vi "VerifyAcqIdle.vi"(8 "error in (no error)":errorcluster, 11 "S4GUI in":refnum<class "S4GUI.lvclass">) -> (0 "error out":errorcluster, 2 "idle":bool, 3 "S4GUI out":refnum<class "S4GUI.lvclass">)   [LabVIEW 2018, in "S4GUI.lvclass"]
uses:
  S4GUI.lvclass
  S4GUI.lvclass/S4GUI.ctl
  Acquisition/Acquisition.lvclass
  Channel/Channel.lvclass
  StateMachine/State Machine.lvclass
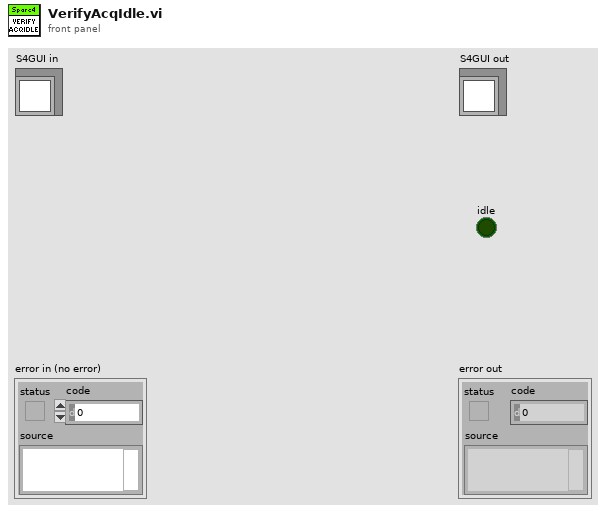
[diagram p1: front panel]
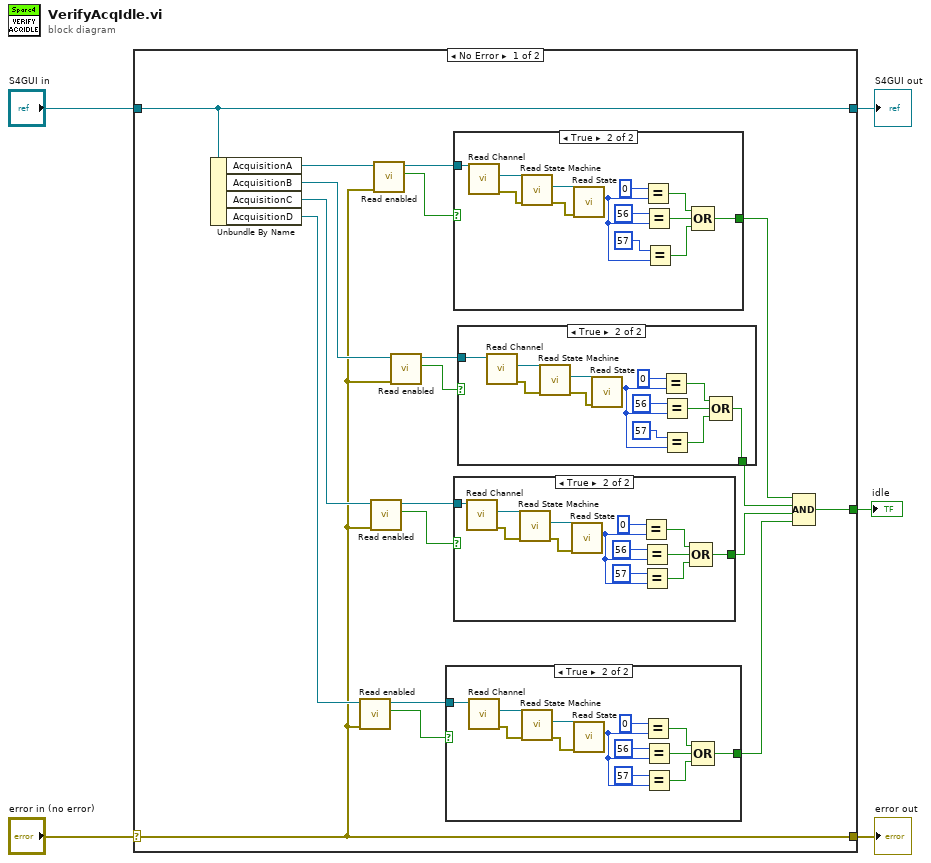
[diagram p0: block diagram]
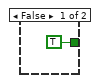
[diagram p2: hidden frame]
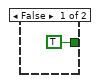
[diagram p3: hidden frame]
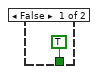
[diagram p4: hidden frame]
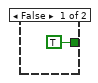
[diagram p5: hidden frame]
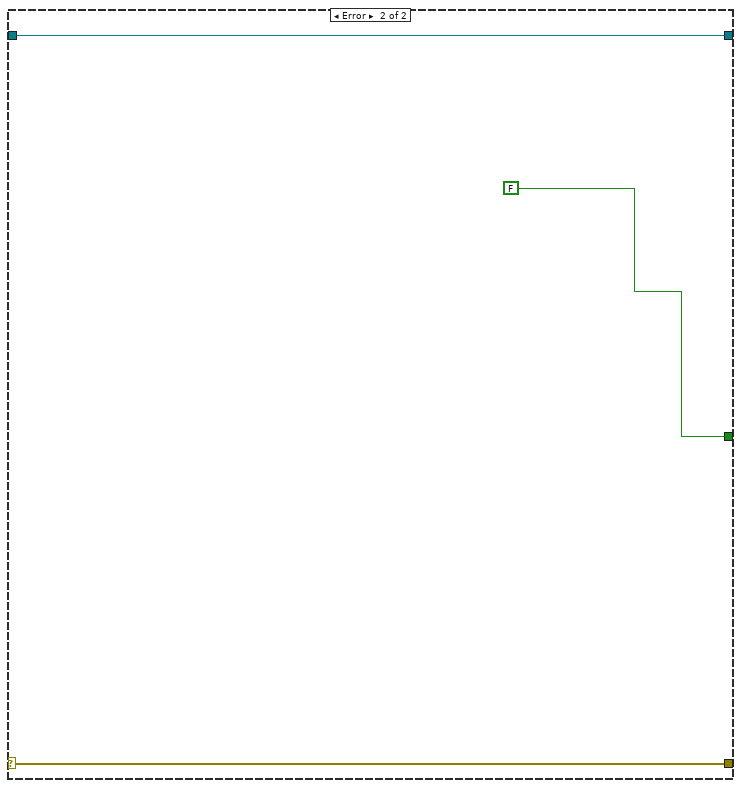
[diagram p6: hidden frame]
diagram:
  n1 = case shown="No Error" "error in (no error)" {
    selector: "error in (no error)" -> [w6 w83]
    tunnel: [w6 w83] -> w4
    tunnel: [w24 w82] -> w2
    tunnel: "S4GUI in" -> [w24 w82]
    tunnel: [w19 FALSE] -> w1
    frame No Error {
      n2 = Unbundle By Name(w24) -> ("AcquisitionA"=w18:refnum<class "Acquisition.lvclass">, "AcquisitionB"=w15:refnum<class "Acquisition.lvclass">, "AcquisitionC"=w12:refnum<class "Acquisition.lvclass">, "AcquisitionD"=w9:refnum<class "Acquisition.lvclass">)
      n3 = call-dynamic "Read enabled.vi"("error in (no error)"=w6, "Server in"=w9) -> ("enabled"=w7:bool, "Server out"=w8:refnum<class "Acquisition.lvclass">)  [unwired: 7 in, 1 out]
      n4 = call-dynamic "Read enabled.vi"("error in (no error)"=w6, "Server in"=w12) -> ("enabled"=w10:bool, "Server out"=w11:refnum<class "Acquisition.lvclass">)  [unwired: 7 in, 1 out]
      n5 = call-dynamic "Read enabled.vi"("error in (no error)"=w6, "Server in"=w18) -> ("enabled"=w16:bool, "Server out"=w17:refnum<class "Acquisition.lvclass">)  [unwired: 7 in, 1 out]
      n6 = call-dynamic "Read enabled.vi"("error in (no error)"=w6, "Server in"=w15) -> ("enabled"=w13:bool, "Server out"=w14:refnum<class "Acquisition.lvclass">)  [unwired: 7 in, 1 out]
      n7 = case shown="True" w7 {
        tunnel: w8 -> [_ w29]
        tunnel: [TRUE w28] -> w20
        frame False {
        }
        frame True {
          n8 = call-dynamic "Read Channel.vi"("Acquisition in"=w29) -> ("error out"=w27:errorcluster, "Channel.lvclass"=w34:refnum<class "Channel.lvclass">)  [unwired: 8 in, 1 out]
          n9 = call-dynamic "Read State Machine.vi"("error in (no error)"=w27, "Device in"=w34) -> ("error out"=w26:errorcluster, "State Machine.lvclass"=w33:refnum<class "State Machine.lvclass">)  [unwired: 7 in, 1 out]
          n10 = call-dynamic "Read State.vi"("error in (no error)"=w26, "State Machine in"=w33) -> ("State"=w32:i32)  [unwired: 7 in, 2 out]
          n11 = Equal?(x=0, y=w32) -> (x = y?=w37:bool)
          n12 = Equal?(x=56, y=w32) -> (x = y?=w36:bool)
          n13 = Equal?(x=57, y=w32) -> (x = y?=w35:bool)
          n14 = Compound Arithmetic op=OR(w37, w36, w35) -> (w28:bool)
        }
      }
      n15 = case shown="True" w16 {
        tunnel: [TRUE w76] -> w23
        tunnel: w17 -> [_ w75]
        frame False {
        }
        frame True {
          n16 = call-dynamic "Read Channel.vi"("Acquisition in"=w75) -> ("error out"=w69:errorcluster, "Channel.lvclass"=w74:refnum<class "Channel.lvclass">)  [unwired: 8 in, 1 out]
          n17 = call-dynamic "Read State Machine.vi"("error in (no error)"=w69, "Device in"=w74) -> ("error out"=w68:errorcluster, "State Machine.lvclass"=w73:refnum<class "State Machine.lvclass">)  [unwired: 7 in, 1 out]
          n18 = call-dynamic "Read State.vi"("error in (no error)"=w68, "State Machine in"=w73) -> ("State"=w72:i32)  [unwired: 7 in, 2 out]
          n19 = Equal?(x=0, y=w72) -> (x = y?=w79:bool)
          n20 = Equal?(x=56, y=w72) -> (x = y?=w78:bool)
          n21 = Equal?(x=57, y=w72) -> (x = y?=w77:bool)
          n22 = Compound Arithmetic op=OR(w79, w78, w77) -> (w76:bool)
        }
      }
      n23 = case shown="True" w10 {
        tunnel: w11 -> [_ w43]
        tunnel: [TRUE w42] -> w21
        frame False {
        }
        frame True {
          n24 = call-dynamic "Read Channel.vi"("Acquisition in"=w43) -> ("error out"=w41:errorcluster, "Channel.lvclass"=w48:refnum<class "Channel.lvclass">)  [unwired: 8 in, 1 out]
          n25 = call-dynamic "Read State Machine.vi"("error in (no error)"=w41, "Device in"=w48) -> ("error out"=w40:errorcluster, "State Machine.lvclass"=w47:refnum<class "State Machine.lvclass">)  [unwired: 7 in, 1 out]
          n26 = call-dynamic "Read State.vi"("error in (no error)"=w40, "State Machine in"=w47) -> ("State"=w46:i32)  [unwired: 7 in, 2 out]
          n27 = Equal?(x=0, y=w46) -> (x = y?=w51:bool)
          n28 = Equal?(x=56, y=w46) -> (x = y?=w50:bool)
          n29 = Equal?(x=57, y=w46) -> (x = y?=w49:bool)
          n30 = Compound Arithmetic op=OR(w51, w50, w49) -> (w42:bool)
        }
      }
      n31 = case shown="True" w13 {
        tunnel: w14 -> [_ w57]
        tunnel: [TRUE w56] -> w22
        frame False {
        }
        frame True {
          n32 = call-dynamic "Read Channel.vi"("Acquisition in"=w57) -> ("error out"=w55:errorcluster, "Channel.lvclass"=w62:refnum<class "Channel.lvclass">)  [unwired: 8 in, 1 out]
          n33 = call-dynamic "Read State Machine.vi"("error in (no error)"=w55, "Device in"=w62) -> ("error out"=w54:errorcluster, "State Machine.lvclass"=w61:refnum<class "State Machine.lvclass">)  [unwired: 7 in, 1 out]
          n34 = call-dynamic "Read State.vi"("error in (no error)"=w54, "State Machine in"=w61) -> ("State"=w60:i32)  [unwired: 7 in, 2 out]
          n35 = Equal?(x=0, y=w60) -> (x = y?=w65:bool)
          n36 = Equal?(x=56, y=w60) -> (x = y?=w64:bool)
          n37 = Equal?(x=57, y=w60) -> (x = y?=w63:bool)
          n38 = Compound Arithmetic op=OR(w65, w64, w63) -> (w56:bool)
        }
      }
      n39 = Compound Arithmetic op=AND(w23, w22, w21, w20) -> (w19:bool)
    }
    frame Error {
    }
  }
  "error out" <- w4
  "S4GUI out" <- w2
  "idle" <- w1
